vi "Dresser DXD Read Error Check.vi"(0 "VISA session":refnum<visa-resource-name>, 1 "DXD Address (1)":T1=1 min=1 max=99 step=1, 5 "Returned String (\"\")":string, 7 "Mode Bit 1 - Error Status Character":enum16{"ACK/NAK", "A/N"}(ring), 9 "Mode Bit 5 - Error Status Character":T2(ring)=enum."No error status character (legacy mode)", 11 "Error In (no error)":errorcluster) -> (4 "dup VISA session":refnum<visa-resource-name>, 6 "Returned String Out":string, 10 "Error":bool, 15 "Error Out":errorcluster)   [LabVIEW 2015]
doc: "This VI reads processes the string returned after a serial buffer read to determine if the Dresser DXD Series pressure transducer returned an error. If there is an error in the buffer, it is placed in the error cluster, otherwise the error produced from reading an empty buffer is cleared. Place the Dresser DXD Error Message.vi after this one to display an error.\n\nWritten by:\nBLOOMY CONTROLS, INC\nWINDSOR, CT 06095, USA\n860-298-9925\nwww.bloomy.com\nV2.0.0\nMay, 2002"
uses:
  Type Defs/DXD Address.ctl
panel:
  # "For instructions on the use of this VI, press Ctrl+H to display the help window and move the mouse over the icon, controls, and indicators"
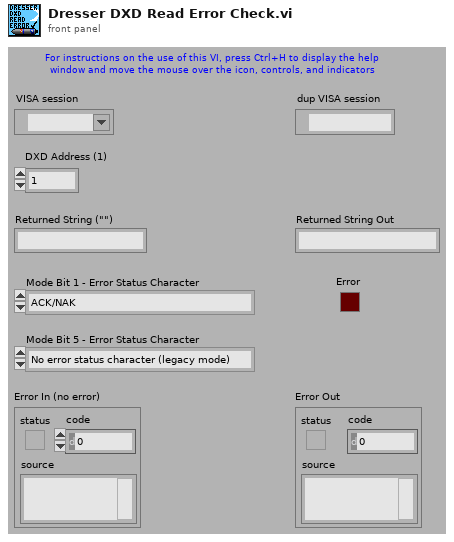
[diagram p1: front panel]
types:
  T1 = typedef "DXD Address.ctl" = i32
  T2 = enum16{"Error status character set in bit 1 is returned", "No error status character (legacy mode)"}
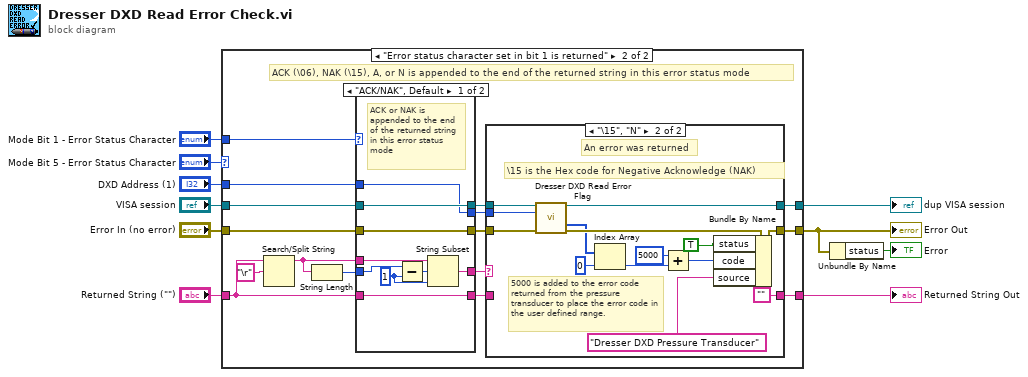
[diagram p0: block diagram]
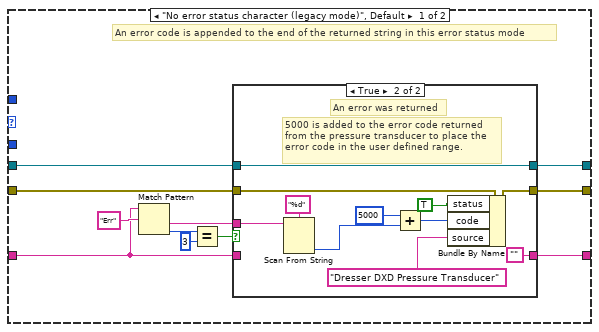
[diagram p2: hidden frame]
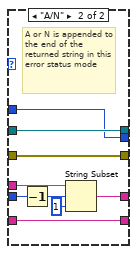
[diagram p5: hidden frame]
diagram:
  n1 = case shown="\"Error status character set in bit 1 is returned\"" "Mode Bit 5 - Error Status Character" {
    tunnel: "Error In (no error)" -> [w18 w51]
    tunnel: "VISA session" -> [w19 w50]
    tunnel: [w14 w38] -> w8
    tunnel: "Returned String (\"\")" -> [w17 w46]
    tunnel: [w16 w36] -> w6
    tunnel: [w15 w37] -> w5
    tunnel: "Mode Bit 1 - Error Status Character" -> [_ w49]
    tunnel: "DXD Address (1)" -> [_ w48]
    frame "No error status character (legacy mode)", Default {
      # "An error code is appended to the end of the returned string in this error status mode"
      n2 = Match Pattern(string=w17, regular expression="Err") -> (after substring=w13:string, offset past match=w12:i32)  [unwired: 1 in, 2 out]
      n3 = Equal?(x=w12, y=3) -> (x = y?=w20:bool)
      n4 = case shown="True" w20 {
        tunnel: w18 -> [w24 w29]
        tunnel: [w24 w28] -> w15
        tunnel: w19 -> [w23 w27]
        tunnel: [w23 w27] -> w14
        tunnel: [w22 ""] -> w16
        tunnel: w17 -> [w22 _]
        tunnel: w13 -> [_ w25]
        frame False {
          # "No error was returned.  Pass the read string out."
        }
        frame True {
          # "5000 is added to the error code returned\nfrom the pressure transducer to place the\nerror code in the user defined range."
          # "An error was returned"
          n5 = Scan From String(format string="%d" ("Format String"), input string=w25) -> (output 1=w32:i32)  [unwired: 3 in, 3 out]
          n6 = Add(x=5000, y=w32) -> (x+y=w31:i32)
          n7 = Bundle By Name(cluster=w29, "status"=TRUE ("Bundle Element"), "code"=w31, "source"="Dresser DXD Pressure Transducer" ("Bundle Element")) -> (w28:errorcluster)
        }
      }
    }
    frame "Error status character set in bit 1 is returned" {
      # "ACK (\\06), NAK (\\15), A, or N is appended to the end of the returned string in this error status mode"
      n8 = Search/Split String(string=w46, search string/char (-)="\r") -> (substring before match=w45:string)  [unwired: 1 in, 2 out]
      n9 = String Length(string=w45) -> (length=w44:i32)
      n10 = case shown="\"ACK/NAK\", Default" w49 {
        tunnel: w51 -> [w72 w80]
        tunnel: w50 -> [w73 w82]
        tunnel: w46 -> [w70 w79]
        tunnel: w48 -> [w71 w81]
        tunnel: w45 -> [w74 w84]
        tunnel: w44 -> [w77 w83]
        tunnel: [w73 w82] -> w43
        tunnel: [w71 w81] -> w42
        tunnel: [w72 w80] -> w41
        tunnel: [w70 w79] -> w40
        tunnel: [w69 w78] -> w39
        frame "ACK/NAK", Default {
          w75 = 1 ("length (rest)")
          # "ACK or NAK is appended to the end of the returned string in this error status mode"
          n11 = Subtract(x=w77, y=w75) -> (x-y=w76:i32)
          n12 = String Subset(string=w74, offset (0)=w76, length (rest)=w75) -> (substring=w69:string)
        }
        frame "A/N" {
          # "A or N is appended to the end of the returned string in this error status mode"
          n13 = Decrement(x=w83) -> (x-1=w86:i32)
          n14 = String Subset(string=w84, offset (0)=w86, length (rest)=1 ("length (rest)")) -> (substring=w78:string)
        }
      }
      n15 = case shown="\"\\15\", \"N\"" w39 {
        tunnel: w41 -> [w54 w62]
        tunnel: [w54 w64] -> w37
        tunnel: w43 -> [w53 w61]
        tunnel: [w53 w60] -> w38
        tunnel: [w52 ""] -> w36
        tunnel: w40 -> [w52 _]
        tunnel: w42 -> [_ w58]
        frame "\u0006", "A", Default {
          # "\\06 is the Hex code for Acknowledge (ACK)"
          # "No error was returned.  Pass the read string out."
        }
        frame "\u0015", "N" {
          # "\\15 is the Hex code for Negative Acknowledge (NAK)"
          # "5000 is added to the error code returned from the pressure transducer to place the error code in the user defined range."
          # "An error was returned"
          n16 = call "Dresser DXD Read Error Flag.vi"("VISA session"=w61, "DXD Address (1)"=w58, "Error In (no error)"=w62) -> ("dup VISA session"=w60:refnum<visa-resource-name>, "Error Codes"=w55:i32[], "Error Out"=w59:errorcluster)  [unwired: 8 in, 2 out]
          n17 = Index Array(array=w55, index=0 ("Index")) -> (element=w56:i32)
          n18 = Add(x=5000, y=w56) -> (x+y=w66:i32)
          n19 = Bundle By Name(cluster=w59, "status"=TRUE ("Bundle Element"), "code"=w66, "source"="Dresser DXD Pressure Transducer" ("Bundle Element")) -> (w64:errorcluster)
        }
      }
    }
  }
  "Error Out" <- w5
  "dup VISA session" <- w8
  "Returned String Out" <- w6
  n20 = Unbundle By Name(w5) -> ("status"=→"Error":bool)
